vi "Update.vi"(8 "Error In":errorcluster, 10 "CommunicationModule":refnum<class "CommunicationModule.lvclass">, 11 "reference in":refnum<class "Logger.lvclass">) -> (0 "Error Out":errorcluster, 3 "reference out":refnum<class "Logger.lvclass">)   [LabVIEW 2024, in "Logger.lvclass"]
uses:
  Logger.lvclass
  Logger.lvclass/Logger.ctl
  CommunicationModule/CommunicationModule.lvclass
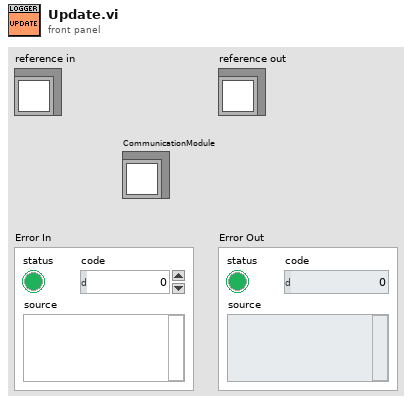
[diagram p1: front panel]
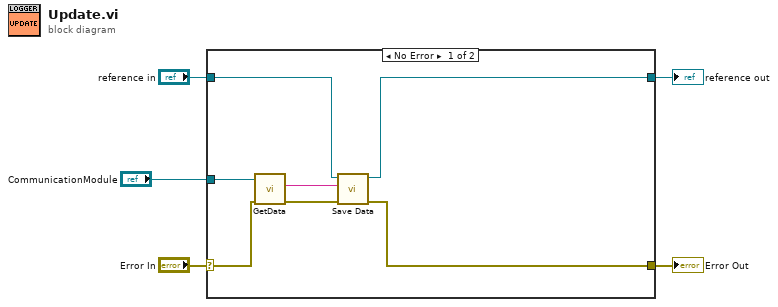
[diagram p0: block diagram]
diagram:
  n1 = case shown="No Error" "Error In" {
    selector: "Error In" -> [w11 w14]
    tunnel: [w9 w14] -> w4
    tunnel: [w7 w13] -> w2
    tunnel: "reference in" -> [w8 w13]
    tunnel: "CommunicationModule" -> [w12 _]
    frame No Error {
      n2 = call-dynamic "GetData.vi"("Error In"=w11, "reference in"=w12) -> ("Error Out"=w10:errorcluster, "Data"=w6:string)  [unwired: 7 in, 1 out]
      n3 = call-dynamic "Save Data.vi"("Error In"=w10, "Data"=w6, "reference in"=w8) -> ("Error Out"=w9:errorcluster, "reference out"=w7:refnum<class "Logger.lvclass">)  [unwired: 7 in]
    }
    frame Error {
    }
  }
  "Error Out" <- w4
  "reference out" <- w2
